vi "UART_SetCommand.vi"(6 "Source Buffer":i32=1250, 7 "EOL Char (Hex)":u8=13 format="%x", 8 "error in (no error)":errorcluster, 9 "Reply Bytes":i32=1250, 10 "Command Byte Array":u8[](array[numeric]) format="%x", 11 "IVI Refnum in":refnum<k15>) -> (0 "error out":errorcluster, 3 "IVI Refnum out":refnum<k15>)   [LabVIEW 2024, in "UART.lvlib"]
doc: "Writes Command Data Byte into uart_source.\nreg0 is the size of the Command Data Byte array\nreg1 is the number of bytes that needs to be received"
uses:
  UART.lvlib
  <instrlib>/niDigital/niDigital.llb/niDigital Write Source Waveform (Broadcast U32).vi
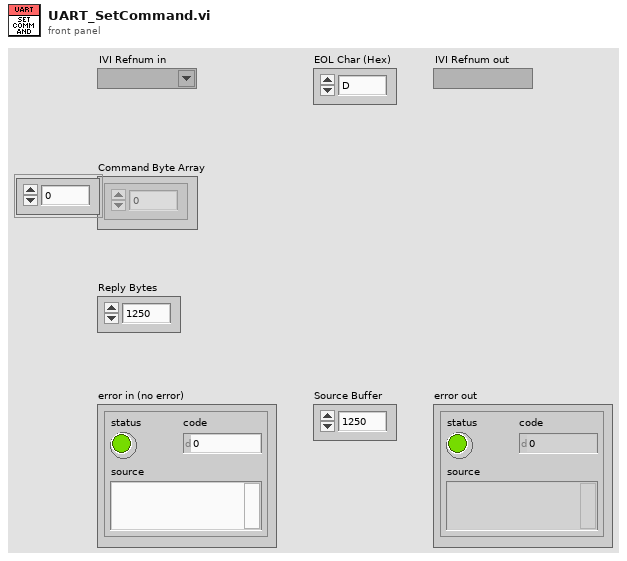
[diagram p1: front panel]
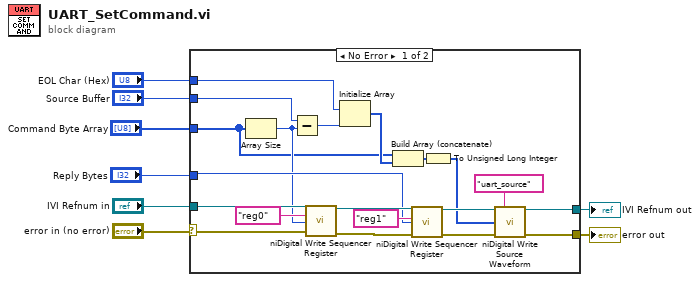
[diagram p0: block diagram]
diagram:
  n1 = case shown="No Error" "error in (no error)" {
    selector: "error in (no error)" -> [w25 w29]
    tunnel: [w28 w29] -> w8
    tunnel: [w27 w30] -> w7
    tunnel: "IVI Refnum in" -> [w26 w30]
    tunnel: "Source Buffer" -> [w13 _]
    tunnel: "EOL Char (Hex)" -> [w12 _]
    tunnel: "Reply Bytes" -> [w11 _]
    tunnel: "Command Byte Array" -> [w9 _]
    frame No Error {
      n2 = Array Size(array=w9) -> (size(s)=w10:i32)
      n3 = Subtract(x=w13, y=w10) -> (x-y=w18:i32)
      n4 = call <instrlib>:"niDigital Write Sequencer Register.vi"("instrument handle"=w26, "sequencer register"="reg0", "value"=w10, "error in"=w25) -> ("instrument handle out"=w24:refnum<k15>, "error out"=w23:errorcluster)  [unwired: 10 in]
      n5 = Initialize Array(w12, w18) -> (w17:u8[])
      n6 = Build Array (concatenate)(w9, w17) -> (w16:u8[])
      n7 = call <instrlib>:"niDigital Write Sequencer Register.vi"("instrument handle"=w24, "sequencer register"="reg1", "value"=w11, "error in"=w23) -> ("instrument handle out"=w21:refnum<k15>, "error out"=w22:errorcluster)  [unwired: 10 in]
      n8 = To Unsigned Long Integer(number=w16) -> (unsigned 32bit integer=w15:u32[])
      n9 = call-poly <instrlib>:"niDigital Write Source Waveform.vi"("instrument handle"=w21, "waveform name"="uart_source", "waveform data"=w15, "error in"=w22) -> ("instrument handle out"=w27:refnum<k15>, "error out"=w28:errorcluster)  [unwired: 10 in]
    }
    frame Error {
    }
  }
  "error out" <- w8
  "IVI Refnum out" <- w7
